vi "Frame Array File.vi"(8 "error in (no error)":errorcluster, 11 "Node Ptr":T3 format="%.0x") -> (0 "error out":errorcluster)   [LabVIEW 2020, in "afdx_custom_device System Explorer.lvlib" / "Implementation.lvlib"]
uses:
  Implementation.lvlib
  <vilib>/NI VeriStand/Custom Device API/Custom Device API.lvlib
  <vilib>/NI VeriStand/Custom Device API/Custom Device Item Ref.ctl
  Types/Configuration File Page Data.ctl
  <vilib>/NI VeriStand/Custom Device Tools/Custom Device Utility Library/Custom Device Utility Library.lvlib
  Types/Browse Button.ctl
  Types/Path Control.ctl
  Scripting/afdx_custom_device Scripting.lvlib
panel:
  in  "Frame Array File":T1
  in  "Refresh":bool
  in  "SHDocVw.IWebBrowser":refnum<k7>(container)
  in  "General Header":cluster{"Section Name":string}={"Section Name"="General Custom Device Settings"}
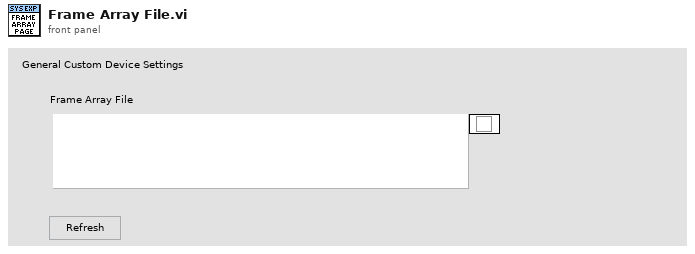
[diagram p1: front panel]
types:
  T1 = typedef "afdx_custom_device System Explorer.lvlib/Implementation.lvlib/Path Control.ctl" = cluster{"file path":path, "Browse":T2}
  T2 = typedef "afdx_custom_device System Explorer.lvlib/Implementation.lvlib/Browse Button.ctl" = bool
  T3 = typedef "Custom Device API.lvlib/Custom Device Item Ref.ctl" = u64
  T4 = typedef "afdx_custom_device System Explorer.lvlib/Implementation.lvlib/Configuration File Page Data.ctl" = cluster{"Parameters":T1, "most recent configuration path":path, "custom device ref":T3, "MD5":string, "configuration path ctl ref":refnum<vi>}
  T5 = typedef "Custom Device API.lvlib/Custom Device Commands.ctl" = enum16{"Default", "Item renamed", "Shutdown", "Dynamic button pressed"}
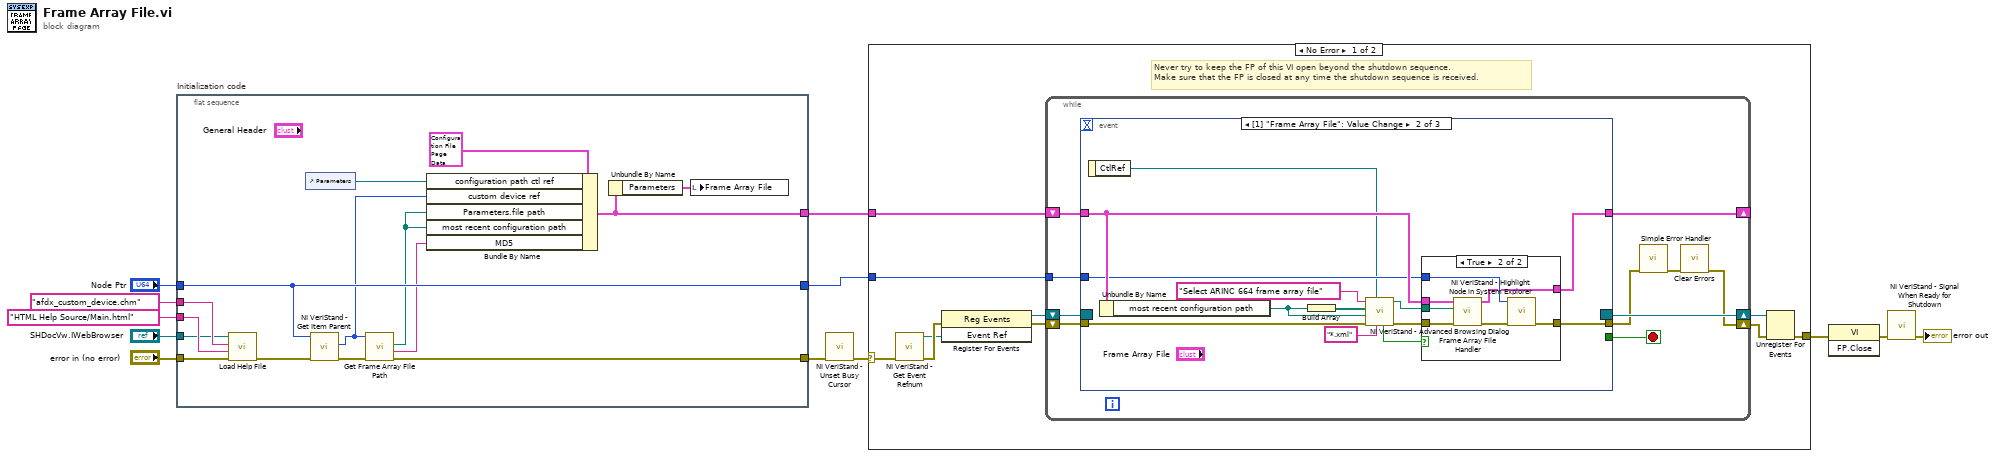
[diagram p0: block diagram]
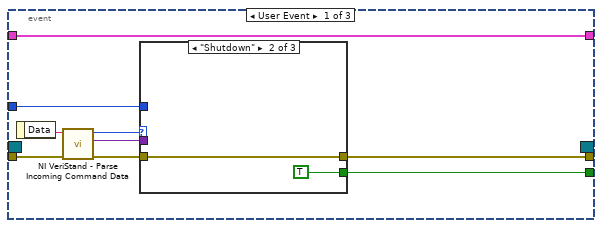
[diagram p2: hidden frame]
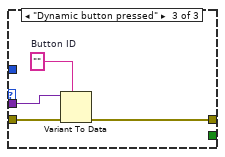
[diagram p4: hidden frame]
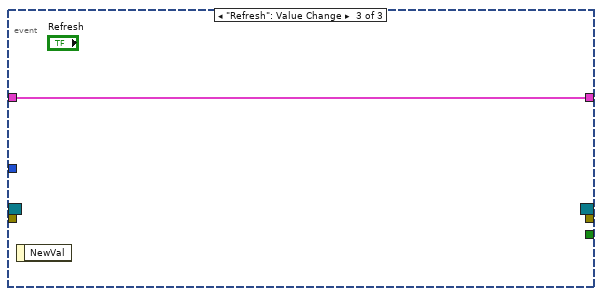
[diagram p6: hidden frame]
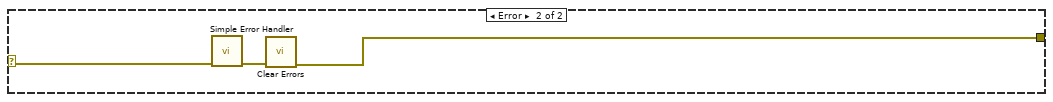
[diagram p7: hidden frame]
diagram:
  n1 = flat-sequence "Initialization code" {
    tunnel: "error in (no error)" -> [w27]
    tunnel: "Node Ptr" -> [w19]
    tunnel: [w15] -> w8
    tunnel: "SHDocVw.IWebBrowser" -> [w23]
    tunnel: "HTML Help Source/Main.html" ("HTML File") -> [w24]
    tunnel: "afdx_custom_device.chm" ("CD_CHM_FileName") -> [w25]
    tunnel: [w21] -> w2
    tunnel: [w19] -> w1
    frame #0 {
      n2 = call "Load Help File.vi"("error in (no error)"=w27, "HTML File to Load"=w24, "Main CHM File"=w25, "Browser"=w23) -> ("error out"=w26:errorcluster)  [unwired: 7 in]
      n3 = control-ref of="Parameters"() -> (w18:refnum<vi>)
      n4 = call <vilib>:"NI VeriStand - Get Item Parent.vi"("error in (no error)"=w26, "Item Ref in"=w19) -> ("error out"=w16:errorcluster, "Parent Ref"=w17:T3)  [unwired: 6 in, 2 out]
      n5 = call "Get Frame Array File Path.vi"("error in"=w16, "custom device ref in"=w17) -> ("error out"=w15:errorcluster, "MD5 checksum"=w14:string, "Frame Array File Path"=w13:path)  [unwired: 5 in, 2 out]
      n6 = Bundle By Name(cluster=T4 {"Parameters"={"file path"=path "", "Browse"=FALSE}, "most recent configuration path"=path "", "custom device ref"=0, "MD5"="", "configuration path ctl ref"=refnum} ("configuration file page data"), "configuration path ctl ref"=w18, "custom device ref"=w17, "Parameters.file path"=w13, "most recent configuration path"=w13, "MD5"=w14) -> (w21:T4)
      n7 = Unbundle By Name(w21) -> ("Parameters"=w20:T1)
      n8 = local write "Frame Array File"(w20) -> ()
    }
  }
  n9 = call <vilib>:"NI VeriStand - Unset Busy Cursor.vi"("error in (no error)"=w8) -> ("error out"=w7:errorcluster)  [unwired: 10 out]
  n10 = case shown="No Error" w7 {
    selector: w7 -> [w29 w89]
    tunnel: [w34 w87] -> w12
    tunnel: w1 -> [w30 _]
    tunnel: w2 -> [w28 _]
    frame No Error {
      # "Never try to keep the FP of this VI open beyond the shutdown sequence.\nMake sure that the FP is closed at any time the shutdown sequence is received."
      n11 = call <vilib>:"NI VeriStand - Get Event Refnum.vi"("error in (no error)"=w29) -> ("error out"=w37:errorcluster, "Event Ref"=w33:refnum<user-event>)  [unwired: 9 out]
      n12 = register-events(error in=w37, w33) -> (reference out=w31:refnum<event-registration>, error out=w32:errorcluster)  [unwired: 1 in]
      n13 = while {
        tunnel: w30 -> [w43]
        shift-right: [w40] -> w35
        shift-left: w32 -> [w46]
        shift-right: [w47] -> w36
        shift-left: w31 -> [w45]
        shift-right: [w38] -> _
        shift-left: w28 -> [w39]
        stop <- w44 stop-if-true
        n14 = event shown="[1] \"Frame Array File\": Value Change" {
          selector: w45 -> [_ _ _]
          dyn-events: [_ _ _] -> w47
          timeout: _ -> [_ _ _]
          tunnel: w46 -> [w56 w76 _]
          tunnel: [w52 _ _] -> w44
          tunnel: [w51 w65 _] -> w42
          tunnel: w43 -> [w50 w67 _]
          tunnel: w39 -> [w48 w68 w86]
          tunnel: [w48 w66 w86] -> w38
          event User Event {
            n15 = event-data() -> ("Data"=w55:string)  [unwired: 1 out]
            n16 = call <vilib>:"NI VeriStand - Parse Incoming Command Data.vi"("error in (no error)"=w56, "Incoming data"=w55) -> ("error out"=w54:errorcluster, "Outgoing data"=w49:variant, "Action"=w53:T5)  [unwired: 7 out]
            n17 = case shown="\"Shutdown\"" w53 {
              tunnel: w54 -> [w57 w58 w63]
              tunnel: [_ TRUE _] -> w52
              tunnel: [w57 w58 w60] -> w51
              tunnel: w50 -> [_ _ _]
              tunnel: w49 -> [_ _ w62]
              frame "Default", Default {
              }
              frame "Shutdown" {
              }
              frame "Dynamic button pressed" {
                w61 = ""  # Button ID
                n18 = Variant To Data(error in=w63, type=w61, Variant=w62) -> (error out=w60:errorcluster)  [unwired: 1 out]
              }
            }
          }
          event Value Change {
            n19 = event-data() -> ("CtlRef"=w64:refnum<vi>)  [unwired: 1 out]
            n20 = Unbundle By Name(w68) -> ("most recent configuration path"=w73:path)
            n21 = Build Array(w73) -> (w74:path[])
            n22 = call <vilib>:"NI VeriStand - Advanced Browsing Dialog.vi"("File Pattern"="*.xml", "CtlRef"=w64, "error in (no error)"=w76, "Most recent path"=w73, "Paths"=w74, "Dialog Title"="Select ARINC 664 frame array file") -> ("error out"=w70:errorcluster, "Selected file"=w69:path, "Valid?"=w71:bool)  [unwired: 2 in, 1 out]
            n23 = case shown="True" w71 {
              tunnel: w70 -> [w77 w85]
              tunnel: w69 -> [_ w84]
              tunnel: w68 -> [w78 w83]
              tunnel: [w77 w81] -> w65
              tunnel: w67 -> [_ w80]
              tunnel: [w78 w79] -> w66
              frame False {
              }
              frame True {
                n24 = call "Frame Array File Handler.vi"("error in"=w85, "selected frame array file"=w84, "configuration file page data"=w83) -> ("error out"=w82:errorcluster, "configuration file page data out"=w79:T4)  [unwired: 7 in]
                n25 = call <vilib>:"NI VeriStand - Highlight Node in System Explorer.vi"("error in (no error)"=w82, "Item Ref in"=w80) -> ("error out"=w81:errorcluster)  [unwired: 8 in, 1 out]
              }
            }
          }
          event "Refresh": Value Change {
            n26 = event-data() -> ()  [unwired: 2 out]
          }
        }
        n27 = call <vilib>:"Simple Error Handler.vi"("error in (no error)"=w42) -> ("error out"=w41:errorcluster)  [unwired: 1 in, 7 out]
        n28 = call <vilib>:"Clear Errors.vi"("error in (no error)"=w41) -> ("error out"=w40:errorcluster)  [unwired: 1 in, 5 out]
      }
      n29 = Unregister For Events(event registration refnum=w36, error in=w35) -> (error out=w34:errorcluster)
    }
    frame Error {
      n30 = call <vilib>:"Simple Error Handler.vi"("error in (no error)"=w89) -> ("error out"=w88:errorcluster)  [unwired: 1 in, 7 out]
      n31 = call <vilib>:"Clear Errors.vi"("error in (no error)"=w88) -> ("error out"=w87:errorcluster)  [unwired: 1 in, 5 out]
    }
  }
  n32 = invoke class="VI" method="FP.Close"(error in=w12) -> (error out=w11:errorcluster)  [unwired: 2 in, 2 out]
  n33 = call <vilib>:"NI VeriStand - Signal When Ready for Shutdown.vi"("error in (no error)"=w11) -> ("error out"=→"error out":errorcluster)  [unwired: 10 out]
